vi "Get Sweep.vi"(0 "Sweep Name":string, 11 "error in (no error)":errorcluster) -> (4 "Variant":variant, 6 "Sweep not found?":bool, 15 "error out":errorcluster)   [LabVIEW 2023, in "RFCalAndFixtureCharact.Common.lvlib"]
uses:
  RFCalAndFixtureCharact.Common.lvlib
  Type Definitions/Dictionary Operation.ctl
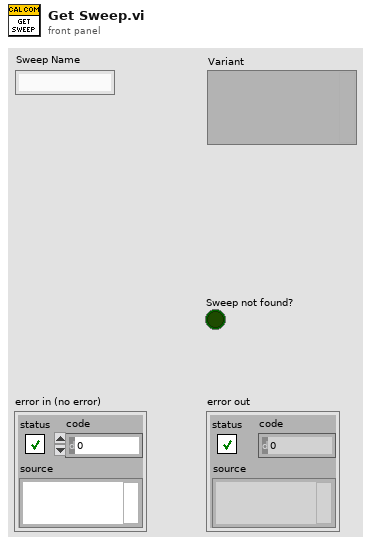
[diagram p1: front panel]
types:
  T1 = typedef "RFCalAndFixtureCharact.Common.lvlib/Dictionary Operation.ctl" = enum16{"Read", "Insert", "Remove", "Clear", "Get All", "Update"}
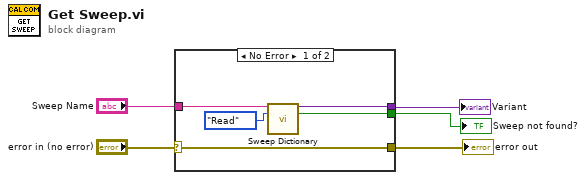
[diagram p0: block diagram]
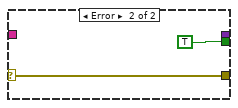
[diagram p2: hidden frame]
diagram:
  n1 = case shown="No Error" "error in (no error)" {
    selector: "error in (no error)" -> [w6 w11]
    tunnel: [w10 _] -> w4
    tunnel: "Sweep Name" -> [w8 _]
    tunnel: [w9 TRUE ("Sweep not found?")] -> w2
    tunnel: [w6 w11] -> w1
    frame No Error {
      n2 = call "Sweep Dictionary.vi"("Sweep name"=w8, "Action"=Dictionary_Operation."Read") -> ("Sweep out"=w10:variant, "Sweep not found / already included"=w9:bool)  [unwired: 11 in, 1 out]
    }
    frame Error {
    }
  }
  "error out" <- w1
  "Variant" <- w4
  "Sweep not found?" <- w2
